vi "CODMn启动命令.vi"(11 "参数":T1={"站号"=21, "量程切换"=enum."AUTO", "控制命令"=0, "模式设置"=enum."待机", "测量间隔"=0} {"站号" items=["CODMn"=21, "总氮"=2, "氨氮"=3]; "控制命令" items=["启动测量"=1, "标样核查"=2, "零点核查"=3, "跨度核查"=4, "空白测试"=5, "平行样测试"=6, "加标回收"=7, "空白校准"=8, "标样校准"=9, "初始化（清洗）"=10, "停止测试"=11, "仪器重启"=12, "校时"=13, "模式设置"=14, "测量间隔设置"=15, "调试"=22, "填充管路"=30, "清洗管路"=31, "清洗反应杯"=32]}) -> (3 "启动命令":cluster{"命令":string, "data":variant})   [LabVIEW 2016, in "斯坦道CODMn新电路板.lvlib"]
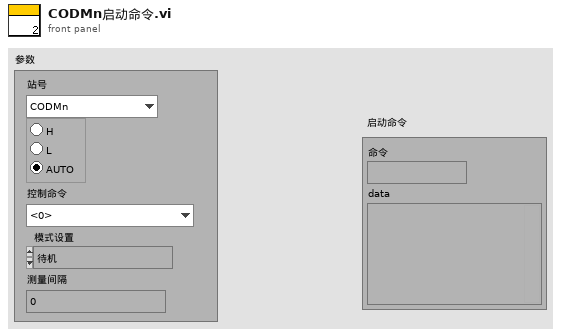
[diagram p1: front panel]
types:
  T1 = cluster{"站号":u16, "量程切换":enum32{"H", "L", "AUTO"}, "控制命令":u16, "模式设置":enum16{"待机", "连续模式", "周期模式", "定点模式", "受控模式", "手动模式"}, "测量间隔":u16}
  T2 = enum16{"待机", "连续模式", "周期模式", "定点模式", "受控模式", "手动模式"}
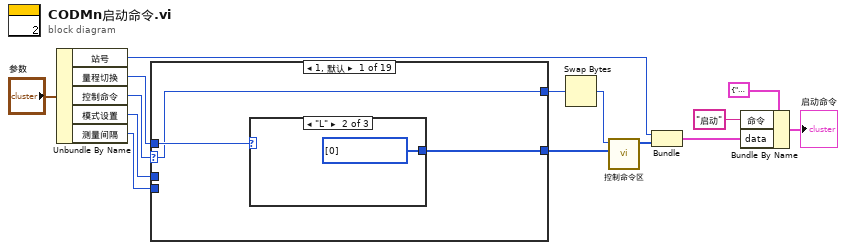
[diagram p0: block diagram]
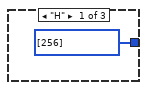
[diagram p2: hidden frame]
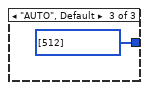
[diagram p3: hidden frame]
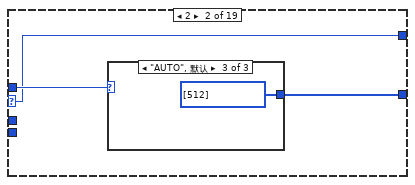
[diagram p4: hidden frame]
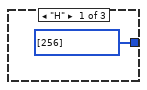
[diagram p5: hidden frame]
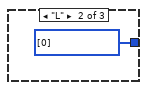
[diagram p6: hidden frame]
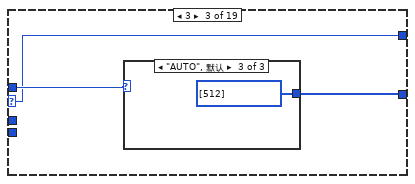
[diagram p7: hidden frame]
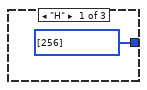
[diagram p8: hidden frame]
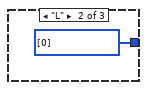
[diagram p9: hidden frame]
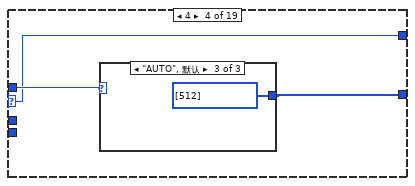
[diagram p10: hidden frame]
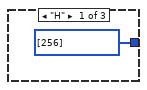
[diagram p11: hidden frame]
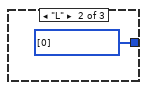
[diagram p12: hidden frame]
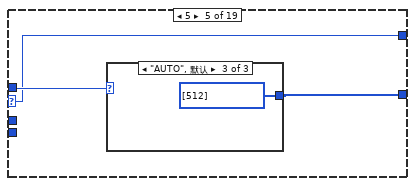
[diagram p13: hidden frame]
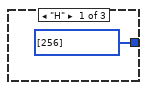
[diagram p14: hidden frame]
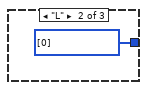
[diagram p15: hidden frame]
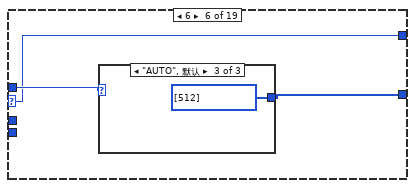
[diagram p16: hidden frame]
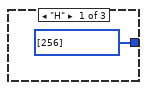
[diagram p17: hidden frame]
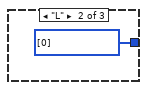
[diagram p18: hidden frame]
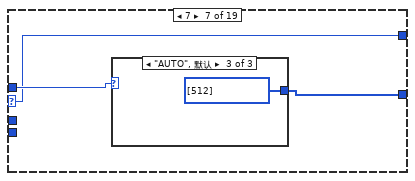
[diagram p19: hidden frame]
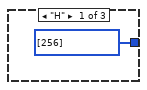
[diagram p20: hidden frame]
diagram:
  n1 = Unbundle By Name("参数") -> ("站号"=w12:u16, "量程切换"=w11:enum32{"H", "L", "AUTO"}, "控制命令"=w10:u16, "模式设置"=w8:T2, "测量间隔"=w9:u16)
  n2 = case shown="1, 默认" w10 {
    selector: w10 -> [w15 w21 w27 w33 w39 w45 w51 w57 w63 w69 w71 w73 w75 w80 w90 w97 w103 w109 w115]
    tunnel: [w17 w23 w28 w34 w40 w47 w53 w59 w65 i32[] [] i32[] [] i32[] [] w76 w82 w92 w96 w102 w107 w114] -> w3
    tunnel: w11 -> [w16 w22 w29 w35 w41 w46 w52 w58 w64 _ _ _ _ _ _ w95 w101 w108 w113]
    tunnel: [w15 w21 w27 w33 w39 w45 w51 w57 w63 w69 w71 w73 w75 w80 w90 w97 w103 w109 w115] -> w2
    tunnel: w9 -> [_ _ _ _ _ _ _ _ _ _ _ _ _ _ w91 _ _ _ _]
    tunnel: w8 -> [_ _ _ _ _ _ _ _ _ _ _ _ _ w81 _ _ _ _ _]
    frame 1, Default {
      n3 = case shown="\"L\"" w16 {
        tunnel: [i32[] [256] i32[] [0] i32[] [512]] -> w17
        frame "H" {
        }
        frame "L" {
        }
        frame "AUTO", Default {
        }
      }
    }
    frame 2 {
      n4 = case shown="\"AUTO\", 默认" w22 {
        tunnel: [i32[] [256] i32[] [0] i32[] [512]] -> w23
        frame "H" {
        }
        frame "L" {
        }
        frame "AUTO", Default {
        }
      }
    }
    frame 3 {
      n5 = case shown="\"AUTO\", 默认" w29 {
        tunnel: [i32[] [256] i32[] [0] i32[] [512]] -> w28
        frame "H" {
        }
        frame "L" {
        }
        frame "AUTO", Default {
        }
      }
    }
    frame 4 {
      n6 = case shown="\"AUTO\", 默认" w35 {
        tunnel: [i32[] [256] i32[] [0] i32[] [512]] -> w34
        frame "H" {
        }
        frame "L" {
        }
        frame "AUTO", Default {
        }
      }
    }
    frame 5 {
      n7 = case shown="\"AUTO\", 默认" w41 {
        tunnel: [i32[] [256] i32[] [0] i32[] [512]] -> w40
        frame "H" {
        }
        frame "L" {
        }
        frame "AUTO", Default {
        }
      }
    }
    frame 6 {
      n8 = case shown="\"AUTO\", 默认" w46 {
        tunnel: [i32[] [256] i32[] [0] i32[] [512]] -> w47
        frame "H" {
        }
        frame "L" {
        }
        frame "AUTO", Default {
        }
      }
    }
    frame 7 {
      n9 = case shown="\"AUTO\", 默认" w52 {
        tunnel: [i32[] [256] i32[] [0] i32[] [512]] -> w53
        frame "H" {
        }
        frame "L" {
        }
        frame "AUTO", Default {
        }
      }
    }
    frame 8 {
      n10 = case shown="\"AUTO\", 默认" w58 {
        tunnel: [i32[] [256] i32[] [0] i32[] [512]] -> w59
        frame "H" {
        }
        frame "L" {
        }
        frame "AUTO", Default {
        }
      }
    }
    frame 9 {
      n11 = case shown="\"AUTO\", 默认" w64 {
        tunnel: [i32[] [256] i32[] [0] i32[] [512]] -> w65
        frame "H" {
        }
        frame "L" {
        }
        frame "AUTO", Default {
        }
      }
    }
    frame 10 {
    }
    frame 11 {
    }
    frame 12 {
    }
    frame 13 {
      n12 = Get Date/Time In Seconds() -> (seconds since 1Jan1904=w79:timestamp)
      n13 = Insert Into Array(array=timestamp[] [] ("数组"), new element=w79) -> (w77:timestamp[])  [unwired: 1 in]
      n14 = call "DateToHex.vi"("DATE"=w77) -> ("数组"=w76:u16[])  [unwired: 10 in]
    }
    frame 14 {
      n15 = case shown="\"定点模式\"" w81 {
        tunnel: [i32[] [0] i32[] [1] i32[] [2] i32[] [3] i32[] [4] i32[] [5]] -> w83
        frame "待机", Default {
        }
        frame "连续模式" {
        }
        frame "周期模式" {
        }
        frame "定点模式" {
        }
        frame "受控模式" {
        }
        frame "手动模式" {
        }
      }
      n16 = call "HexToWord.vi"("数组"=w83) -> ("WORD"=w82:u16[])  [unwired: 10 in]
    }
    frame 15 {
      n17 = Replace Array Subset(array=i32[] [0], new element=w91) -> (w93:i32[])  [unwired: 1 in]
      n18 = call "HexToWord.vi"("数组"=w93) -> ("WORD"=w92:u16[])  [unwired: 10 in]
    }
    frame 22 {
      n19 = case shown="\"L\"" w95 {
        tunnel: [i32[] [256] i32[] [0] i32[] [512]] -> w96
        frame "H" {
        }
        frame "L" {
        }
        frame "AUTO", Default {
        }
      }
    }
    frame 30 {
      n20 = case shown="\"L\"" w101 {
        tunnel: [i32[] [256] i32[] [0] i32[] [512]] -> w102
        frame "H" {
        }
        frame "L" {
        }
        frame "AUTO", Default {
        }
      }
    }
    frame 31 {
      n21 = case shown="\"L\"" w108 {
        tunnel: [i32[] [256] i32[] [0] i32[] [512]] -> w107
        frame "H" {
        }
        frame "L" {
        }
        frame "AUTO", Default {
        }
      }
    }
    frame 32 {
      n22 = case shown="\"L\"" w113 {
        tunnel: [i32[] [256] i32[] [0] i32[] [512]] -> w114
        frame "H" {
        }
        frame "L" {
        }
        frame "AUTO", Default {
        }
      }
    }
  }
  n23 = Swap Bytes(anything=w2) -> (byte swapped=w1:u16)
  n24 = call "控制命令区.vi"("控制命令参数"=w3, "控制命令"=w1) -> ("控制命令"=w7:u16[])  [unwired: 9 in]
  n25 = Bundle("站号"=w12, "控制命令"=w7) -> (w4:cluster{"站号":u16, "控制命令":u16[]})  [unwired: 1 in]
  n26 = Bundle By Name(cluster=cluster{"命令":string, "data":variant} {"命令"="", "data"=variant} ("元素"), "命令"="启动", "data"=w4) -> (→"启动命令":cluster{"命令":string, "data":variant})
